vi "Declare Liveliness Wrapper.vi"(8 "error in (no error)":errorcluster, 10 "Key Expression":string="labviewnode", 11 "Session in":u64) -> (0 "error out":errorcluster, 3 "Liveliness Token":u64)   [LabVIEW 2021, in "Zenoh.lvclass"]
uses:
  Zenoh.lvclass
  typedef/Zenoh Errors.ctl
  SubVIs/Add Zenoh Error Core.vi
  Zenoh.lvclass/Zenoh.ctl
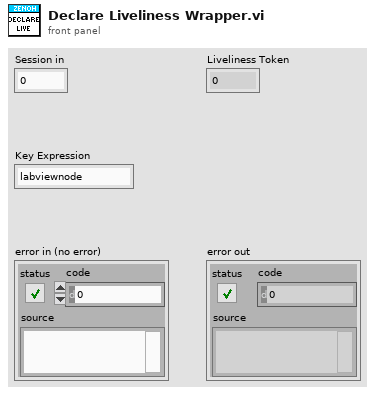
[diagram p1: front panel]
types:
  T1 = typedef "Zenoh.lvclass/Zenoh Errors.ctl" = enum16{"Open Session Error", "Open Subscription Error", "Declare Liveliness", "Query Keys", "File Error", "JSON Error", "Zenoh Runtime"}
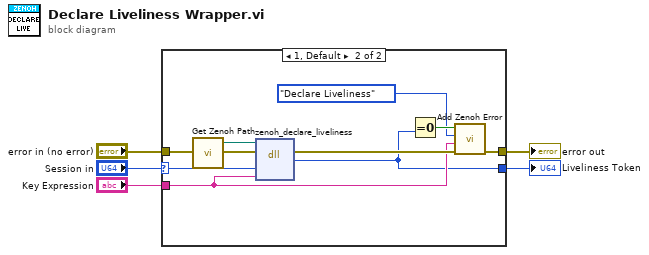
[diagram p0: block diagram]
diagram:
  n1 = case shown="1, Default" "Session in" {
    selector: "Session in" -> [_ w8]
    tunnel: [w6 w15] -> w5
    tunnel: "error in (no error)" -> [w6 w11]
    tunnel: [_ w7] -> w3
    tunnel: "Key Expression" -> [_ w9]
    frame 0 {
    }
    frame 1, Default {
      n2 = call "Get Zenoh Path.vi"() -> ("Library Path"=w12:path)  [unwired: 4 in]
      n3 = dll-call lib="C:/Program Files/CIF_Foundation/Libraries/zenoh_lv_wrapper.dll" fn="zenoh_declare_liveliness"(path in=w12, error in=w11, "session_prt"=w8, "key_expr"=w9) -> (error out=w10:errorcluster, "LivelinessToken"=w7:u64)  [unwired: 3 in, 1 out]
      n4 = Equal To 0?(x=w7) -> (x = 0?=w14:bool)
      n5 = call "Add Zenoh Error.vi"("error in (no error)"=w10, "String to Append"=w9, "Error"=Zenoh_Errors."Declare Liveliness", "Insert Error"=w14) -> ("error out"=w15:errorcluster)  [unwired: 7 in]
    }
  }
  "error out" <- w5
  "Liveliness Token" <- w3
